vi "document_module.vi"() -> ()   [LabVIEW 2018]
panel:
  in  "MAIN_MINIMIZE":bool
  out "MAIN_STATUS_TRANS":bool caption="CAUTION!"
  out "MAIN_INFO_USER":string
  in  "MAIN_CLOSE":bool
  out "MAIN_INFO_NOTE":string caption="String"
  in  "MAIN_TAB":T1(tab)
  in  "reg_delete":bool
  in  "reg_find":bool
  in  "reg_register":bool
  in  "reg_MANF     :":string caption="MANF     :"
  in  "reg_ATA      :":string caption="ATA      :"
  in  "reg_PN       :":string caption="PN       :"
  in  "reg_REV. DATE:":string caption="REV. DATE:"
  in  "reg_REVISION :":string caption="REVISION :"
  in  "reg_TITLE    :":string caption="TITLE    :"
  in  "reg_DOC. NO  :":string caption="DOC. NO  :"
  out "2D Picture":picture
  in  "trans_submit":bool
  in  "trans_EVALUATION":string caption="EVALUATION"
  in  "trans_Search Document Number":string caption="Search Document Number"
  in  "trans_TITLE    :":string caption="TITLE    :"
  in  "trans_REVISION :":string caption="REVISION :"
  in  "trans_REV. DATE:":string caption="REV. DATE:"
  in  "trans_PN       :":string caption="PN       :"
  in  "trans_ATA      :":string caption="ATA      :"
  in  "trans_MANF     :":string caption="MANF     :"
  out "2D Picture 2":picture
  in  "str_print":bool caption="Button 3"
  in  "str_Search Document Number":string caption="Search Document Number"
  in  "str_LOC":string caption="LOC"
  in  "str_MANF     :":string caption="MANF     :"
  in  "str_ATA      :":string caption="ATA      :"
  in  "str_PN       :":string caption="PN       :"
  in  "str_REV. DATE:":string caption="REV. DATE:"
  in  "str_REVISION :":string caption="REVISION :"
  in  "str_TITLE    :":string caption="TITLE    :"
  # "DOCUMENT MODULE"
  # "DOCUMENT REGISTRATION"
  # "DOCUMENT TRANSFER"
  # "DOCUMENT STORE"
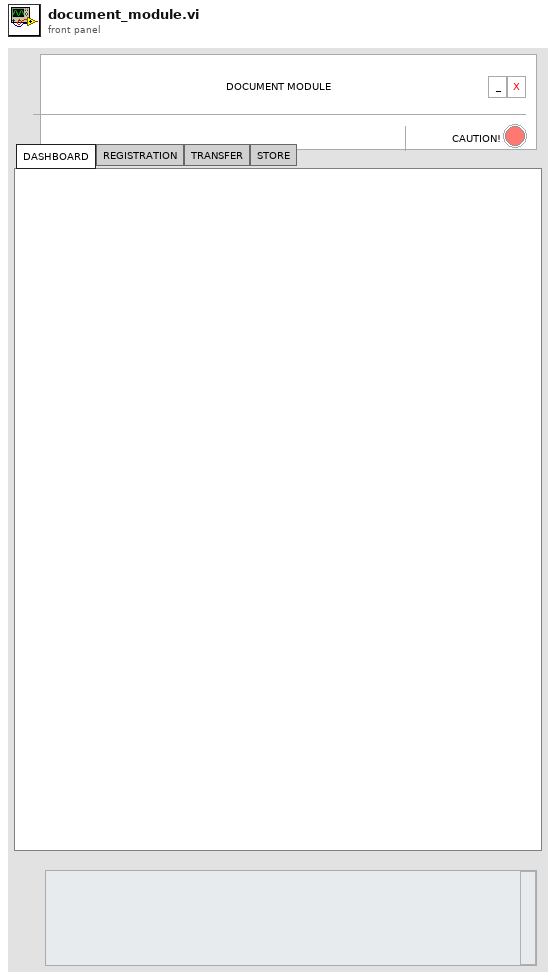
[diagram p1: front panel]
types:
  T1 = enum32{"DASHBOARD", "REGISTRATION", "TRANSFER", "STORE"}
  T2 = enum32{"Size Tabs To Contents", "Size All Tabs to Largest Tab", "Fixed Tab Size"}
  T3 = enum32{"Invalid", "Standard", "Closed", "Hidden", "Minimized", "Maximized"}
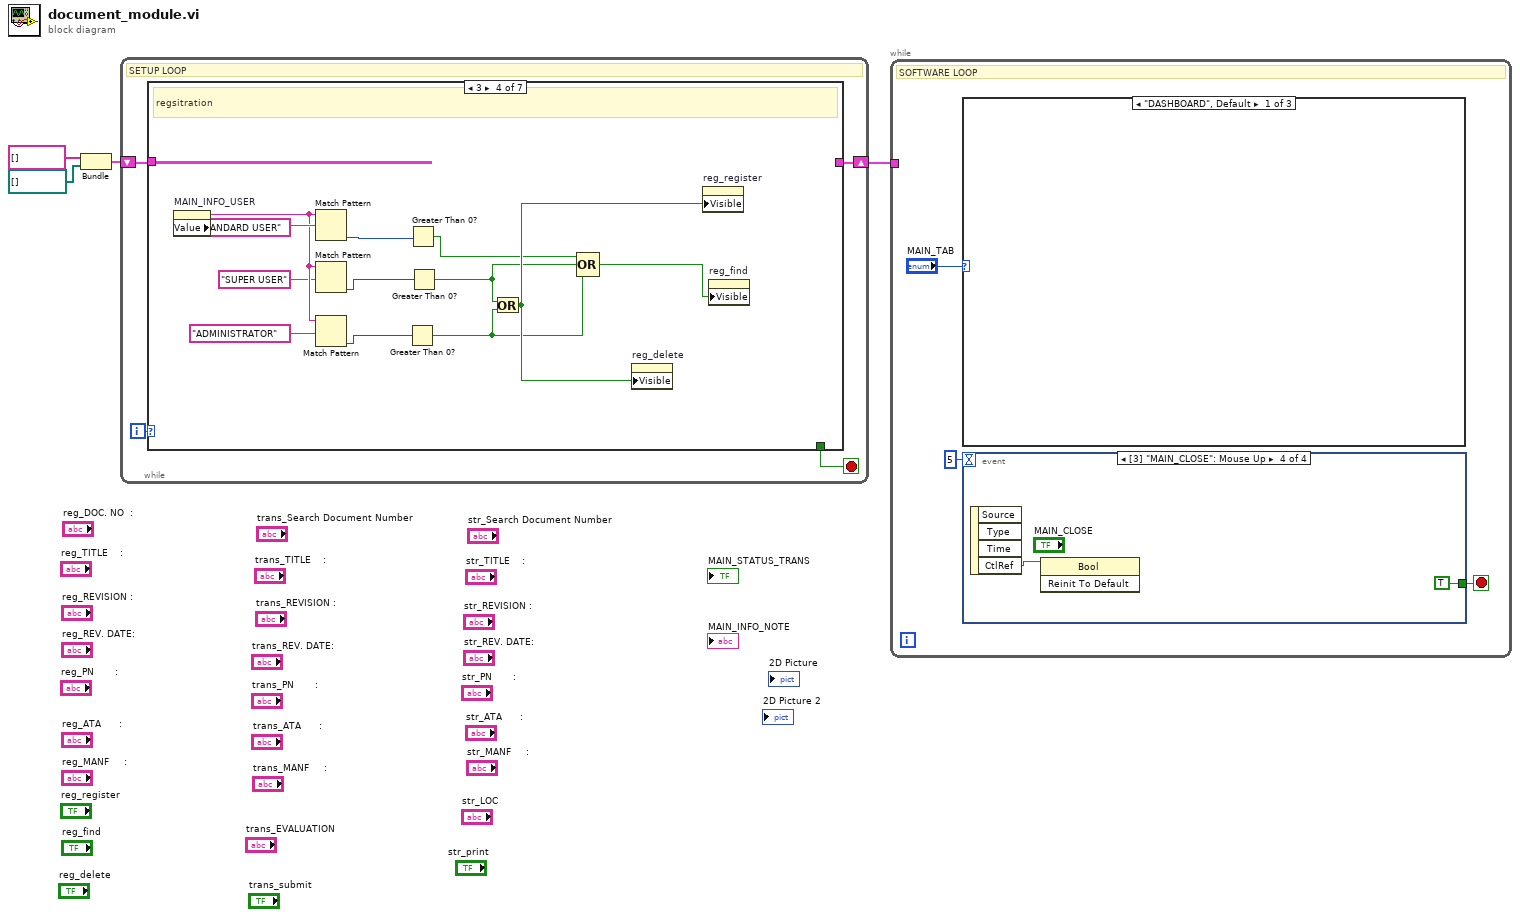
[diagram p0: block diagram]
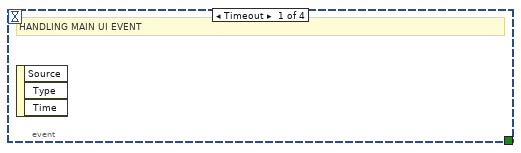
[diagram p2: hidden frame]
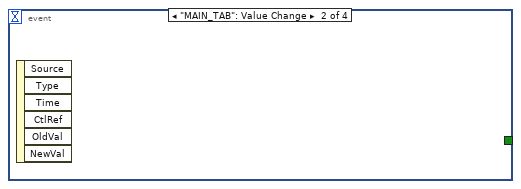
[diagram p3: hidden frame]
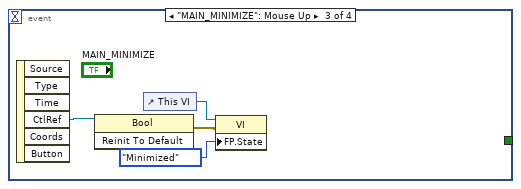
[diagram p4: hidden frame]
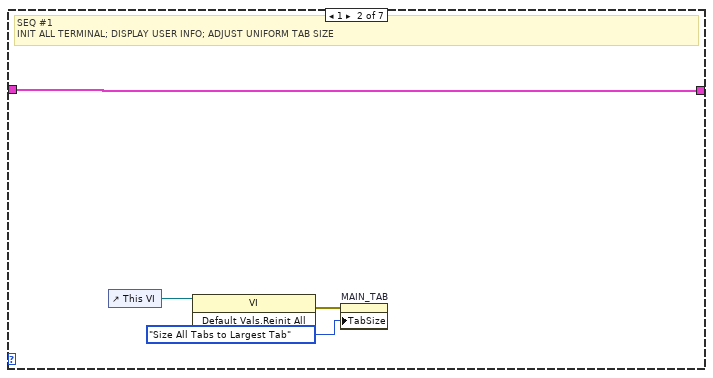
[diagram p8: hidden frame]
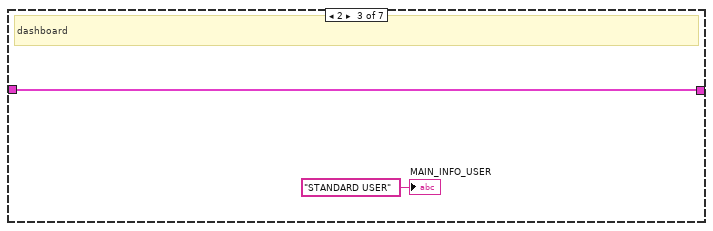
[diagram p9: hidden frame]
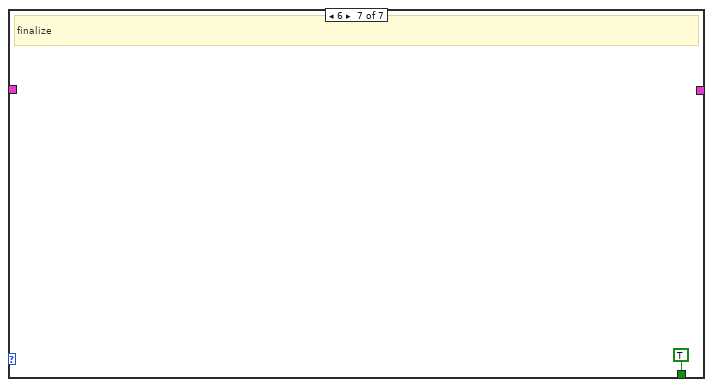
[diagram p12: hidden frame]
diagram:
  n1 = Bundle(string[] [], path[] []) -> (w1:cluster{string[], path[]})  [unwired: 1 in]
  n2 = while {
    shift-right: [w7] -> w2
    shift-left: w1 -> [w6]
    i -> [w8]
    stop <- w5 stop-if-true
    # "SETUP LOOP"
    n3 = case shown="3" w8 {
      tunnel: w6 -> [w9 w12 w15 _ _ _ _]
      tunnel: [w9 w12 w15 _ _ _ _] -> w7
      tunnel: [_ _ _ _ _ _ TRUE] -> w5
      frame 0, Default {
        # "SEQ #0\nCOMMAND LINE ARGUMENTS"
      }
      frame 1 {
        # "SEQ #1\nINIT ALL TERMINAL; DISPLAY USER INFO; ADJUST UNIFORM TAB SIZE"
        n4 = control-ref of="This VI"() -> (w13:refnum<vi>)
        n5 = invoke class="VI" method="Default Vals.Reinit All"(reference=w13) -> (error out=w11:errorcluster)  [unwired: 2 in, 2 out]
        n6 = property on="MAIN_TAB" class="TabCtl (strict)"(error in=w11, "TabSize"=T2."Size All Tabs to Largest Tab" ("Tab Size")) -> ()  [unwired: 1 in, 2 out]
      }
      frame 2 {
        # "dashboard"
        "MAIN_INFO_USER" <- "STANDARD USER" ("MAIN_INFO_USER")
      }
      frame 3 {
        # "regsitration"
        n7 = property on="MAIN_INFO_USER" class="Str"() -> ("Value"=w25:string)  [unwired: 2 in, 2 out]
        n8 = Match Pattern(string=w25, regular expression="STANDARD USER") -> (offset past match=w26:i32)  [unwired: 1 in, 3 out]
        n9 = Match Pattern(string=w25, regular expression="SUPER USER") -> (offset past match=w22:i32)  [unwired: 1 in, 3 out]
        n10 = Match Pattern(string=w25, regular expression="ADMINISTRATOR") -> (offset past match=w21:i32)  [unwired: 1 in, 3 out]
        n11 = Greater Than 0?(x=w21) -> (x > 0?=w19:bool)
        n12 = Greater Than 0?(x=w26) -> (x > 0?=w17:bool)
        n13 = Greater Than 0?(x=w22) -> (x > 0?=w18:bool)
        n14 = Or(x=w18, y=w19) -> (x .or. y?=w20:bool)
        n15 = Compound Arithmetic op=OR(w17, w18, w19) -> (w16:bool)
        n16 = property on="reg_delete" class="Bool"("Visible"=w20) -> ()  [unwired: 2 in, 2 out]
        n17 = property on="reg_register" class="Bool"("Visible"=w20) -> ()  [unwired: 2 in, 2 out]
        n18 = property on="reg_find" class="Bool"("Visible"=w16) -> ()  [unwired: 2 in, 2 out]
      }
      frame 4 {
        # "transfer"
      }
      frame 5 {
        # "store"
      }
      frame 6 {
        # "finalize"
      }
    }
  }
  n19 = while {
    tunnel: w2 -> [_]
    stop <- w29 stop-if-true
    # "SOFTWARE LOOP"
    n20 = case shown="\"DASHBOARD\", Default" "MAIN_TAB" {
      frame "DASHBOARD", Default {
      }
      frame "REGISTRATION" {
      }
      frame "TRANSFER" {
      }
    }
    n21 = event shown="[3] \"MAIN_CLOSE\": Mouse Up" {
      selector: _ -> [_ _ _ _]
      dyn-events: _ -> [_ _ _ _]
      timeout: 5 -> [_ _ _ _]
      tunnel: [_ _ _ TRUE] -> w29
      event Timeout {
        # "HANDLING MAIN UI EVENT"
        n22 = event-data() -> ()  [unwired: 1 in, 3 out]
      }
      event "MAIN_TAB": Value Change {
        n23 = event-data() -> ()  [unwired: 1 in, 6 out]
      }
      event "MAIN_MINIMIZE": Mouse Up {
        n24 = event-data() -> ("CtlRef"=w33:refnum<vi>)  [unwired: 1 in, 5 out]
        n25 = invoke class="Bool" method="Reinit To Default"(reference=w33) -> (error out=w32:errorcluster)  [unwired: 2 in, 2 out]
        n26 = control-ref of="This VI"() -> (w35:refnum<vi>)
        n27 = property class="VI"(reference=w35, error in=w32, "FP.State"=T3."Minimized" ("Front Panel Window:State")) -> ()  [unwired: 2 out]
      }
      event "MAIN_CLOSE": Mouse Up {
        n28 = event-data() -> ("CtlRef"=w37:refnum<vi>)  [unwired: 1 in, 3 out]
        n29 = invoke class="Bool" method="Reinit To Default"(reference=w37) -> ()  [unwired: 2 in, 3 out]
      }
    }
  }
